vi "InitClimber.vi"   [LabVIEW 2020]
doc: "This VI initializes devices related to the climber subsytem."
uses:
  <vilib>/Rock Robotics/WPI/Solenoid/WPI_SolenoidChannel.ctl
  <vilib>/Rock Robotics/WPI/ThirdParty/Phoenix-LabVIEW/Motor Controller/Controls/CTRE_Phoenix_MotorControl_TalonFXInvertType.ctl
  <vilib>/Rock Robotics/WPI/ThirdParty/Phoenix-LabVIEW/Motor Controller/Controls/CTRE_Phoenix_MotorControl_NeutralMode.ctl
  <vilib>/Rock Robotics/WPI/ThirdParty/Phoenix-LabVIEW/Motor Controller/Controls/CTRE_Phoenix_MotorControl_SupplyCurrentLimitConfiguration.ctl
  <vilib>/Rock Robotics/WPI/ThirdParty/Phoenix-LabVIEW/Motor Controller/Controls/CTRE_Phoenix_MotorControl_FeedbackDevice_TalonFX.ctl
  <vilib>/Rock Robotics/WPI/Solenoid/WPI_SolenoidOpenDouble.vi
  refnumbers.vi
types:
  T1 = typedef "CTRE_Phoenix_MotorControl_FeedbackDevice_TalonFX.ctl" = i8
  T2 = typedef "CTRE_Phoenix_MotorControl_SupplyCurrentLimitConfiguration.ctl" = cluster{"Enable?":bool, "Current Limit":dbl, "Threshold Current":dbl, "Threshold Time":dbl}
  T3 = typedef "CTRE_Phoenix_MotorControl_NeutralMode.ctl" = enum8{"EEPROMSetting", "Override to Coast", "Override to Brake"}
  T4 = typedef "CTRE_Phoenix_MotorControl_TalonFXInvertType.ctl" = enum16{"Counter-Clockwise", "Clockwise"}
  T5 = typedef "WPI_SolenoidChannel.ctl" = enum8{"Solenoid 0", "Solenoid 1", "Solenoid 2", "Solenoid 3", "Solenoid 4", "Solenoid 5", "Solenoid 6", "Solenoid 7", "Solenoid 8", "Solenoid 9", "Solenoid 10", "Solenoid 11", "Solenoid 12", "Solenoid 13", "Solenoid 14", "Solenoid 15", "Invalid"}
  T6 = typedef "WPI_MotorControlDeviceRef.ctl" = cluster{"DeviceStatus":errorcluster, "Type":T7, "PWM":cluster{"PWM Channel":T8, "DeadBand":T9}, "CAN":cluster{"Device Number":u8, "SetOutput VI Ref":variant, "GetOutput VI Ref":variant, "Enable VI Ref":variant, "Disable VI Ref":variant, "Data":variant}, "Invert":bool, "DIO PWM":cluster{"PWM \"Enable\" Channel":T8, "DIOChannel":T10, "PWM Rate":dbl}}
  T7 = typedef "WPI_MotorControlType.ctl" = enum16{"PWM", "CAN", "DIO PWM"}
  T8 = typedef "FPGA_DIOPWMChannel.ctl" = enum8{"PWM 0", "PWM 1", "PWM 2", "PWM 3", "PWM 4", "PWM 5", "PWM 6", "PWM 7", "PWM 8", "PWM 9", "PWM MXP 0", "PWM MXP 1", "PWM MXP 2", "PWM MXP 3", "PWM MXP 4", "PWM MXP 5", "PWM MXP 6", "PWM MXP 7", "PWM MXP 8", "PWM MXP 9", "Invalid"}
  T9 = typedef "WPI_PWMDeadband.ctl" = cluster{"Name":string, "maxPositivePwm":i32, "minPositivePwm":i32, "centerPwm":i32, "maxNegativePwm":i32, "minNegativePwm":i32, "angularRange":u16}
  T10 = typedef "FPGA_DIOChannel.ctl" = enum8{"DIO 0", "DIO 1", "DIO 2", "DIO 3", "DIO 4", "DIO 5", "DIO 6", "DIO 7", "DIO 8", "DIO 9", "DIO MXP 0", "DIO MXP 1", "DIO MXP 2", "DIO MXP 3", "DIO MXP 4", "DIO MXP 5", "DIO MXP 6", "DIO MXP 7", "DIO MXP 8", "DIO MXP 9", "DIO MXP 10", "DIO MXP 11", "DIO MXP 12", "DIO MXP 13", "DIO MXP 14", "DIO MXP 15", "SPI Port CS1", "SPI Port CS2", "SPI Port CS3", "SPI Port MISO", "SPI Port MOSI", "Invalid"}
  T11 = typedef "WPI_SolenoidDevRef.ctl" = cluster{"DevStatus":errorcluster, "Pneumatics Control Module":u8, "Forward Solenoid Channel":T5, "Reverse Solenoid Channel":T5}
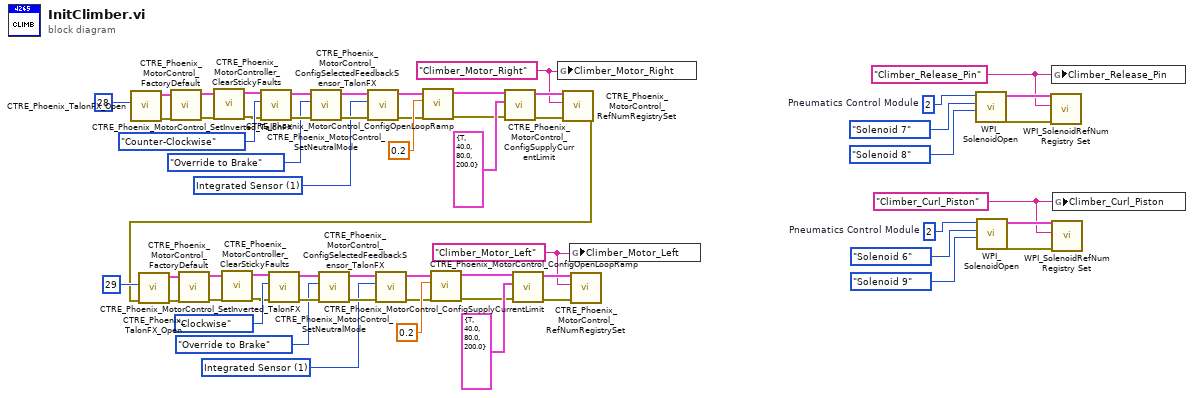
[diagram p0: block diagram]
diagram:
  w10 = T1 1 items=["Integrated Sensor"=1, "Sensor Sum (S0 + S1)"=9, "Sensor Difference (D0 - D1)"=10, "Remote Source 0"=11, "Remote Source 1"=12, "None"=14, "Software Emulated"=15] ("Talon FX Feedback Device")
  w14 = "Climber_Motor_Left" ("refnum name")
  w33 = T1 1 items=["Integrated Sensor"=1, "Sensor Sum (S0 + S1)"=9, "Sensor Difference (D0 - D1)"=10, "Remote Source 0"=11, "Remote Source 1"=12, "None"=14, "Software Emulated"=15] ("Talon FX Feedback Device")
  w37 = "Climber_Motor_Right" ("refnum name")
  w49 = "Climber_Curl_Piston" ("refnum name")
  w53 = u8 2  # Pneumatics Control Module
  w55 = "Climber_Release_Pin" ("refnum name")
  w59 = u8 2  # Pneumatics Control Module
  n1 = call <vilib>:"CTRE_Phoenix_TalonFX_Open.vi"("Device Number"=u8 28) -> ("error out"=w47:errorcluster, "PhoenixMotorControlDevRef"=w46:T6)  [unwired: 9 in]
  n2 = call <vilib>:"CTRE_Phoenix_MotorControl_FactoryDefault.vi"("error in"=w47, "PhoenixMotorControlDevRef"=w46) -> ("error out"=w30:errorcluster, "PhoenixMotorControlDevRef"=w29:T6)  [unwired: 8 in]
  n3 = call <vilib>:"CTRE_Phoenix_MotorController_ClearStickyFaults.vi"("error in"=w30, "PhoenixMotorControlDevRef"=w29) -> ("error out"=w27:errorcluster, "PhoenixMotorControlDevRef"=w28:T6)  [unwired: 8 in]
  n4 = call <vilib>:"CTRE_Phoenix_MotorControl_SetInverted_TalonFX.vi"("error in (no error)"=w27, "Invert Type"=CTRE_Phoenix_MotorControl_TalonFXInvertType."Counter-Clockwise", "PhoenixMotorControlDevRef"=w28) -> ("error out"=w44:errorcluster, "PhoenixMotorControlDevRef"=w43:T6)  [unwired: 7 in]
  n5 = call <vilib>:"CTRE_Phoenix_MotorControl_SetNeutralMode.vi"("error in (no error)"=w44, "Motor Control Neutral Mode"=CTRE_Phoenix_MotorControl_NeutralMode."Override to Brake", "PhoenixMotorControlDevRef"=w43) -> ("error out"=w34:errorcluster, "PhoenixMotorControlDevRef"=w35:T6)  [unwired: 7 in]
  n6 = call <vilib>:"CTRE_Phoenix_MotorControl_ConfigSelectedFeedbackSensor_TalonFX.vi"("error in (no error)"=w34, "Talon FX Feedback Device"=w33, "PhoenixMotorControlDevRef"=w35) -> ("error out"=w31:errorcluster, "PhoenixMotorControlDevRef"=w32:T6)  [unwired: 7 in]
  n7 = call <vilib>:"CTRE_Phoenix_MotorControl_ConfigOpenLoopRamp.vi"("error in (no error)"=w31, "secondsFromNeutralToFull"=0.2, "PhoenixMotorControlDevRef"=w32) -> ("error out"=w25:errorcluster, "PhoenixMotorControlDevRef"=w26:T6)  [unwired: 7 in]
  n8 = call <vilib>:"CTRE_Phoenix_MotorControl_ConfigSupplyCurrentLimit.vi"("error in (no error)"=w25, "Supply Current Limit Configuration"=T2 {"Enable?"=TRUE, "Current Limit"=40.0, "Threshold Current"=80.0, "Threshold Time"=200.0}, "PhoenixMotorControlDevRef"=w26) -> ("error out"=w39:errorcluster, "PhoenixMotorControlDevRef"=w38:T6)  [unwired: 7 in]
  n9 = global write "refnumbers.vi" "Climber_Motor_Right"(w37) -> ()
  n10 = call <vilib>:"CTRE_Phoenix_MotorControl_RefNumRegistrySet.vi"("error in (no error)"=w39, "refnum name"=w37, "PhoenixMotorControlDevRef"=w38) -> ("error out"=w1:errorcluster)  [unwired: 7 in, 1 out]
  n11 = call <vilib>:"CTRE_Phoenix_TalonFX_Open.vi"("error in"=w1, "Device Number"=u8 29) -> ("error out"=w24:errorcluster, "PhoenixMotorControlDevRef"=w23:T6)  [unwired: 8 in]
  n12 = call <vilib>:"CTRE_Phoenix_MotorControl_FactoryDefault.vi"("error in"=w24, "PhoenixMotorControlDevRef"=w23) -> ("error out"=w7:errorcluster, "PhoenixMotorControlDevRef"=w6:T6)  [unwired: 8 in]
  n13 = call <vilib>:"CTRE_Phoenix_MotorController_ClearStickyFaults.vi"("error in"=w7, "PhoenixMotorControlDevRef"=w6) -> ("error out"=w4:errorcluster, "PhoenixMotorControlDevRef"=w5:T6)  [unwired: 8 in]
  n14 = call <vilib>:"CTRE_Phoenix_MotorControl_SetInverted_TalonFX.vi"("error in (no error)"=w4, "Invert Type"=CTRE_Phoenix_MotorControl_TalonFXInvertType."Clockwise", "PhoenixMotorControlDevRef"=w5) -> ("error out"=w21:errorcluster, "PhoenixMotorControlDevRef"=w20:T6)  [unwired: 7 in]
  n15 = call <vilib>:"CTRE_Phoenix_MotorControl_SetNeutralMode.vi"("error in (no error)"=w21, "Motor Control Neutral Mode"=CTRE_Phoenix_MotorControl_NeutralMode."Override to Brake", "PhoenixMotorControlDevRef"=w20) -> ("error out"=w11:errorcluster, "PhoenixMotorControlDevRef"=w12:T6)  [unwired: 7 in]
  n16 = call <vilib>:"CTRE_Phoenix_MotorControl_ConfigSelectedFeedbackSensor_TalonFX.vi"("error in (no error)"=w11, "Talon FX Feedback Device"=w10, "PhoenixMotorControlDevRef"=w12) -> ("error out"=w8:errorcluster, "PhoenixMotorControlDevRef"=w9:T6)  [unwired: 7 in]
  n17 = call <vilib>:"CTRE_Phoenix_MotorControl_ConfigOpenLoopRamp.vi"("error in (no error)"=w8, "secondsFromNeutralToFull"=0.2, "PhoenixMotorControlDevRef"=w9) -> ("error out"=w2:errorcluster, "PhoenixMotorControlDevRef"=w3:T6)  [unwired: 7 in]
  n18 = call <vilib>:"CTRE_Phoenix_MotorControl_ConfigSupplyCurrentLimit.vi"("error in (no error)"=w2, "Supply Current Limit Configuration"=T2 {"Enable?"=TRUE, "Current Limit"=40.0, "Threshold Current"=80.0, "Threshold Time"=200.0}, "PhoenixMotorControlDevRef"=w3) -> ("error out"=w16:errorcluster, "PhoenixMotorControlDevRef"=w15:T6)  [unwired: 7 in]
  n19 = global write "refnumbers.vi" "Climber_Motor_Left"(w14) -> ()
  n20 = call <vilib>:"CTRE_Phoenix_MotorControl_RefNumRegistrySet.vi"("error in (no error)"=w16, "refnum name"=w14, "PhoenixMotorControlDevRef"=w15) -> ()  [unwired: 7 in, 2 out]
  n21 = call-poly <vilib>:"WPI_SolenoidOpen.vi"("Reverse Solenoid Channel"=WPI_SolenoidChannel."Solenoid 8", "Forward Solenoid Channel"=WPI_SolenoidChannel."Solenoid 7", "Pneumatics Device (def)"=w59) -> ("error out"=w56:errorcluster, "SolenoidDevRef"=w57:T11)  [unwired: 7 in]
  n22 = call-poly <vilib>:"WPI_SolenoidOpen.vi"("Reverse Solenoid Channel"=WPI_SolenoidChannel."Solenoid 9", "Forward Solenoid Channel"=WPI_SolenoidChannel."Solenoid 6", "Pneumatics Device (def)"=w53) -> ("error out"=w50:errorcluster, "SolenoidDevRef"=w51:T11)  [unwired: 7 in]
  n23 = call <vilib>:"WPI_SolenoidRefNum Registry Set.vi"("error in (no error)"=w56, "refnum name"=w55, "SolenoidDevRef"=w57) -> ()  [unwired: 7 in, 2 out]
  n24 = global write "refnumbers.vi" "Climber_Release_Pin"(w55) -> ()
  n25 = call <vilib>:"WPI_SolenoidRefNum Registry Set.vi"("error in (no error)"=w50, "refnum name"=w49, "SolenoidDevRef"=w51) -> ()  [unwired: 7 in, 2 out]
  n26 = global write "refnumbers.vi" "Climber_Curl_Piston"(w49) -> ()
